vi "Master Setup CheckPath.vi"(8 "error in":errorcluster, 11 "filepath":path) -> (0 "error out":errorcluster, 1 "pla available?":bool, 2 "pmgr available?":bool, 3 "match substring":string)   [LabVIEW 2017]
doc: "Check the path is *.pmgr or *.pla?"
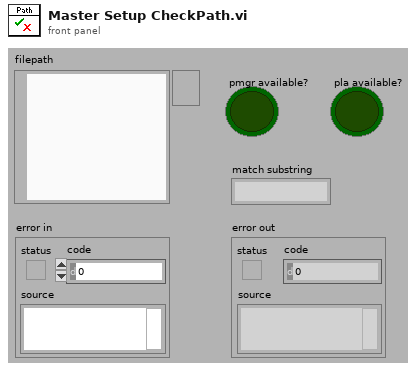
[diagram p1: front panel]
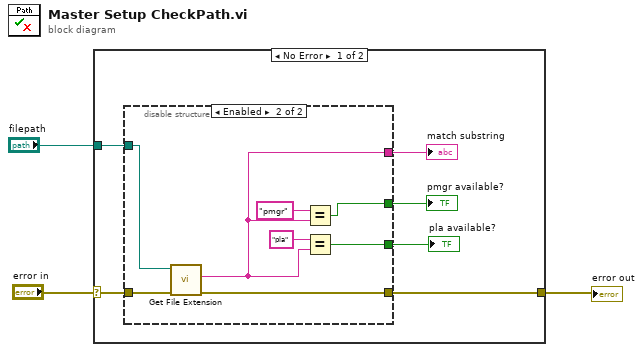
[diagram p0: block diagram]
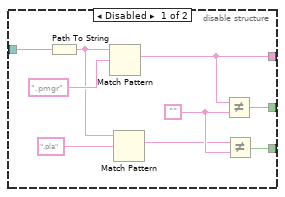
[diagram p2: hidden frame]
diagram:
  n1 = case shown="No Error" "error in" {
    selector: "error in" -> [w5 w27]
    tunnel: [w4 w27] -> w2
    tunnel: "filepath" -> [w9 _]
    frame No Error {
      n2 = disable-structure shown="Enabled" {
        disable-tunnel: w9 -> [w17 w24]
        disable-tunnel: [w14 w19] -> w8
        disable-tunnel: [w11 w21] -> w7
        disable-tunnel: [w10 w20] -> w6
        disable-tunnel: w5 -> [_ w26]
        disable-tunnel: [_ w25] -> w4
        frame Disabled {
          w13 = ""
          n3 = Path To String(path=w17) -> (string=w16:string)
          n4 = Match Pattern(string=w16, regular expression=".pmgr" ("search string")) -> (match substring=w14:string)  [unwired: 1 in, 3 out]
          n5 = Match Pattern(string=w16, regular expression=".pla") -> (match substring=w12:string)  [unwired: 1 in, 3 out]
          n6 = Not Equal?(x=w14, y=w13) -> (x != y?=w11:bool)
          n7 = Not Equal?(x=w12, y=w13) -> (x != y?=w10:bool)
        }
        frame Enabled {
          n8 = call <vilib>:"Get File Extension.vi"("error in (no error)"=w26, "file"=w24) -> ("error out"=w25:errorcluster, "lowercase file extension"=w19:string)  [unwired: 5 in, 3 out]
          n9 = Equal?(x="pmgr", y=w19) -> (x = y?=w21:bool)
          n10 = Equal?(x="pla", y=w19) -> (x = y?=w20:bool)
        }
      }
      "match substring" <- w8
      "pmgr available?" <- w7
      "pla available?" <- w6
    }
    frame Error {
    }
  }
  "error out" <- w2
